vi "lightsMotorsFansNames.vi"() -> ()   [LabVIEW 2019]
uses:
  <vilib>/Instr/_visa.llb/VISA Set IO Buffer Mask.ctl
  <vilib>/Instr/_visa.llb/VISA Configure Serial Port (Instr).vi
panel:
  in  "zone 1 inlet":i32
  in  "zone 1 return":i32
  in  "Fans":i32
  in  "zone 2 inlet":i32
  in  "zone 3 inlet":i32
  in  "zone 2 return":i32
  in  "zone 1 co2":i32
  in  "Light 3":i32
  in  "fresh air":i32
  in  "zone 2 co2":i32
  in  "Light 1":i32
  in  "zone 3 return":i32
  in  "Light 2":i32
  in  "zone 3 co2":i32
  in  "VISA- Arduino Mega":refnum<visa-resource-name>
  in  "stop":bool
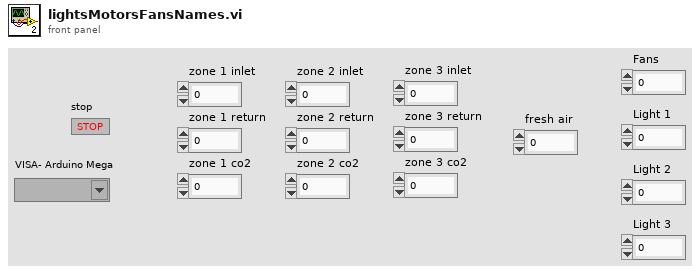
[diagram p1: front panel]
types:
  T1 = typedef "VISA Set IO Buffer Mask.ctl" = u16
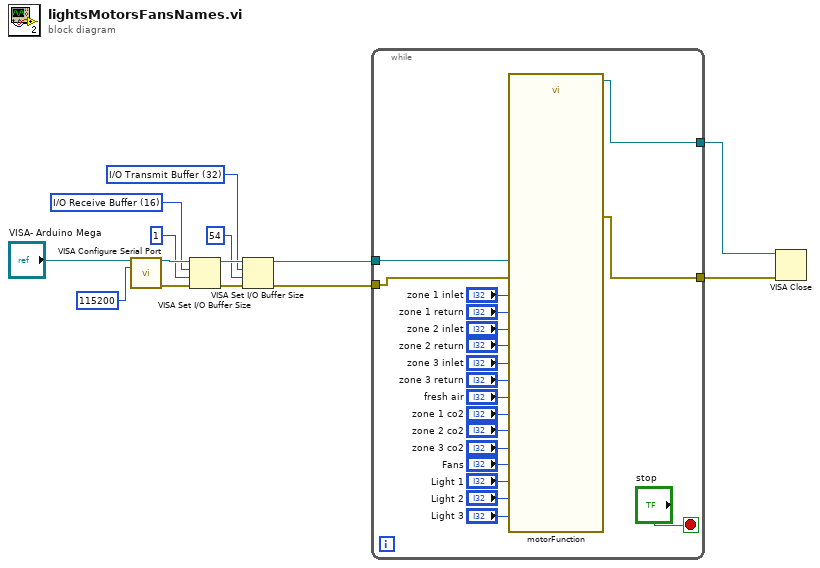
[diagram p0: block diagram]
diagram:
  w3 = T1 32 items=["I/O Receive Buffer"=16, "I/O Transmit Buffer"=32, "I/O Receive and Transmit Buffer"=48] ("Mask")
  w6 = T1 16 items=["I/O Receive Buffer"=16, "I/O Transmit Buffer"=32, "I/O Receive and Transmit Buffer"=48] ("Mask")
  n1 = call-poly "VISA Configure Serial Port"("VISA resource name"="VISA- Arduino Mega", "baud rate (115200)"=u32 115200 ("baud rate (9600)")) -> ("VISA resource name out"=w9:refnum<visa-resource-name>, "error out"=w8:errorcluster)  [unwired: 12 in]
  n2 = VISA Set I/O Buffer Size(VISA resource name=w9, mask (16)=w6, size (4096)=u32 1, error in (no error)=w8) -> (VISA resource name out=w4:refnum<visa-resource-name>, error out=w5:errorcluster)
  n3 = VISA Set I/O Buffer Size(VISA resource name=w4, mask (16)=w3, size (4096)=u32 54, error in (no error)=w5) -> (VISA resource name out=w13:refnum<visa-resource-name>, error out=w12:errorcluster)
  n4 = while {
    tunnel: w12 -> [w32]
    tunnel: w13 -> [w31]
    tunnel: [w30] -> w11
    tunnel: [w29] -> w10
    stop <- "stop" stop-if-true
    n5 = call "motorFunction.vi"("VISA Refnum in"=w31, "zone 3 co2"="zone 3 co2", "Light 2"="Light 2", "zone 3 return"="zone 3 return", "Light 1"="Light 1", "zone 2 co2"="zone 2 co2", "fresh air"="fresh air", "error in (no error)"=w32, "Light 3"="Light 3", "zone 1 co2"="zone 1 co2", "zone 2 return"="zone 2 return", "zone 3 inlet"="zone 3 inlet", "zone 2 inlet"="zone 2 inlet", "Fans"="Fans", "zone 1 return"="zone 1 return", "zone 1 inlet"="zone 1 inlet") -> ("VISA Refnum out"=w29:refnum<visa-resource-name>, "error out"=w30:errorcluster)  [unwired: 10 in]
  }
  n6 = VISA Close(VISA resource name=w10, error in (no error)=w11) -> ()  [unwired: 1 out]
